vi "open dataset.vi"(9 "old dataset":T1) -> (1 "new dataset":T1)   [LabVIEW 2025]
panel:
  # "Load or Save dataset. \nDataset includes raw data, data names, scales, show/hide indices parameters."
  # "On: Scale parameters defined by 'scaling' function will be used."
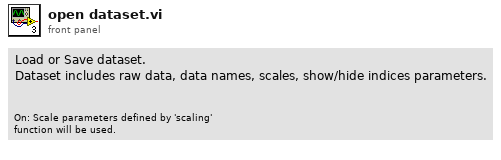
[diagram p1: front panel]
types:
  T1 = cluster{"data cluster":cluster{"all data":dbl[][]}[], "Scale":u16, "scale matrix":dbl[][], "universal y-scale":dbl, "data names":string[], "new dataset?":bool, "show files 2":cluster{"String":string, "Boolean":bool, "begin":u32, "length":u32, "y weight":dbl}[]}
  T2 = enum16{"Left Button", "Center Button", "Right Button", "Window Close"}
  T3 = cluster{"String":string, "Boolean":bool, "begin":u32, "length":u32, "y weight":dbl}[]
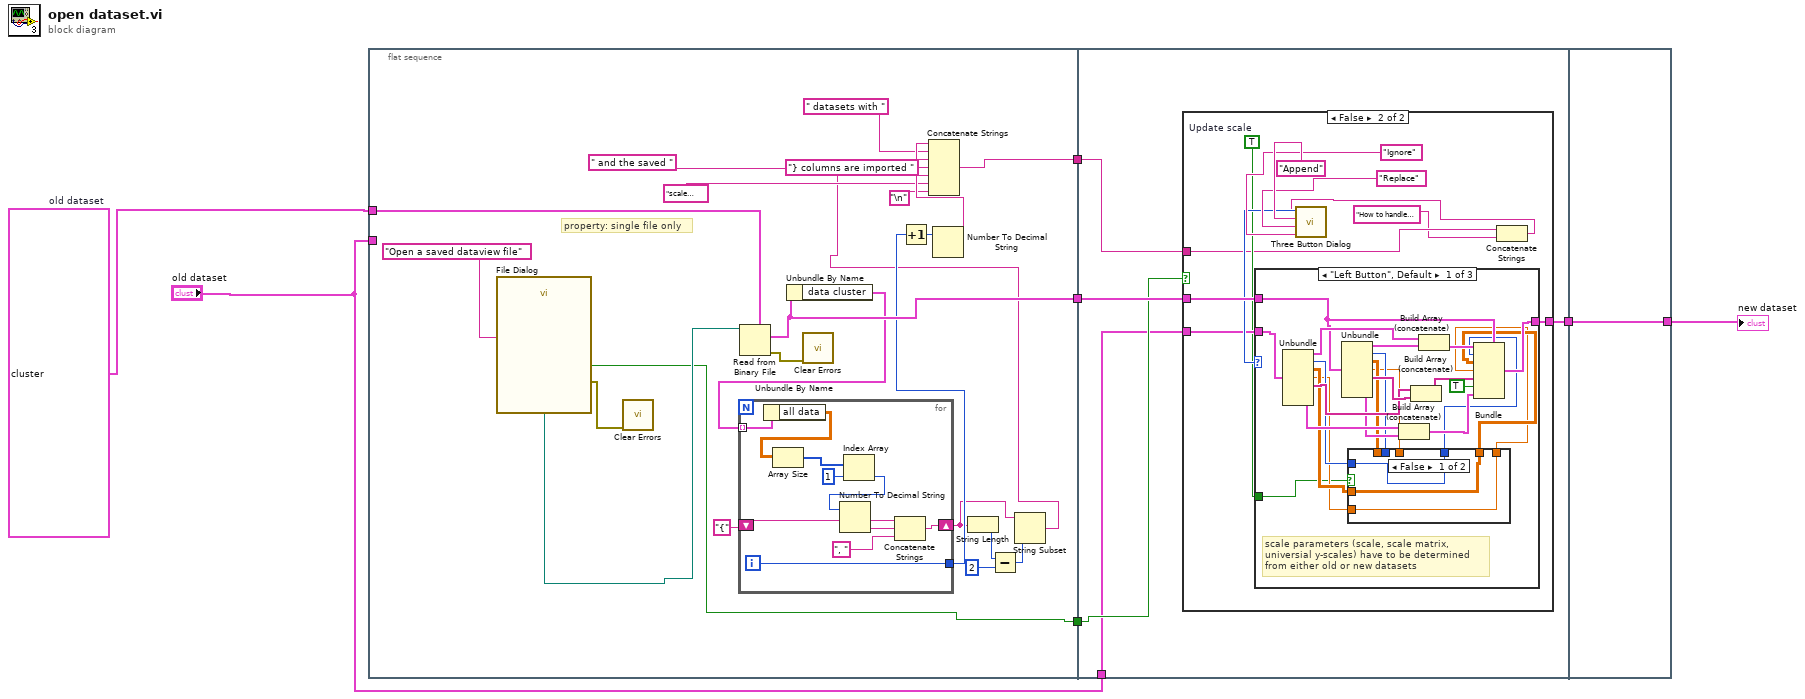
[diagram p0: block diagram]
diagram:
  w6 = T1 {"data cluster"=[{"all data"=array60x36[2160 elements]}], "Scale"=0, "scale matrix"=[], "universal y-scale"=1.0, "data names"=["FGT512para_PPMS_Hsweep_170K3.dat"], "new dataset?"=TRUE, "show files 2"=[]}  # old dataset
  n1 = flat-sequence {
    tunnel: [w19] -> w5
    tunnel: [w28] -> w4
    tunnel: "old dataset" -> [_]
    tunnel: w6 -> [w27]
    tunnel: [w20] -> w2
    tunnel: w5 -> [w45]
    tunnel: "old dataset" -> [w42]
    tunnel: [w44] -> w3
    tunnel: w4 -> [w43]
    tunnel: w2 -> [w41]
    tunnel: [w89] -> w1
    tunnel: w3 -> [w89]
    frame #0 {
      # "property: single file only"
      n2 = call "File Dialog"("prompt"="Open a saved dataview file") -> ("selected path"=w29:path, "cancelled"=w28:bool, "error out"=w30:errorcluster)  [unwired: 11 in, 1 out]
      n3 = call <vilib>:"Clear Errors.vi"("error in (no error)"=w30) -> ()  [unwired: 5 in, 2 out]
      n4 = Read from Binary File(5:w27, 11:w29) -> (0:w26:errorcluster, 2:w19:T1)  [unwired: 4 in, 2 out]
      n5 = Unbundle By Name(w19) -> ("data cluster"=w18:cluster{"all data":dbl[][]}[])
      n6 = for {
        tunnel: w18 -> [w38] mode=indexing
        tunnel: [w36] -> w17
        shift-right: [w31] -> w12
        shift-left: "{" -> [w34]
        i -> [w36]
        n7 = Unbundle By Name(w38) -> ("all data"=w37:dbl[][])
        n8 = Array Size(array=w37) -> (size(s)=w40:i32[])
        n9 = Index Array(array=w40, index=1) -> (element=w35:i32)
        n10 = Number To Decimal String(number=w35) -> (decimal integer string=w33:string)  [unwired: 1 in]
        n11 = Concatenate Strings(w34, w33, ", " ("string")) -> (w31:string)
      }
      n12 = call <vilib>:"Clear Errors.vi"("error in (no error)"=w26) -> ()  [unwired: 5 in, 2 out]
      n13 = Increment(x=w17) -> (x+1=w16:i32)
      n14 = Number To Decimal String(number=w16) -> (decimal integer string=w24:string)  [unwired: 1 in]
      n15 = String Length(string=w12) -> (length=w10:i32)
      n16 = Subtract(x=w10, y=2) -> (x-y=w8:i32)
      n17 = String Subset(string=w12, length (rest)=w8) -> (substring=w11:string)  [unwired: 1 in]
      n18 = Concatenate Strings(w24, " datasets with " ("string"), w11, "} columns are imported " ("string"), " and the saved " ("Center Button Text (\"No\")"), "scale parameters will be used." ("string"), "\n") -> (w20:string)
    }
    frame #1 {
      n19 = case shown="False" w43 {
        tunnel: w45 -> [_ w54]
        tunnel: [w46 w53] -> w44
        tunnel: w42 -> [w46 w51]
        tunnel: w41 -> [_ w48]
        frame True {
        }
        frame False {
          w49 = TRUE  # Update scale
          n20 = Concatenate Strings(w48, "How to handle the loaded datasets?" ("message")) -> (w50:string)
          n21 = call <vilib>:"Three Button Dialog.vi"("Right Button Text (\"Cancel\")"="Ignore" ("Right Button Text (\"Cancel\")"), "Center Button Text (\"No\")"="Replace" ("Center Button Text (\"No\")"), "Left Button Text (\"Yes\")"="Append" ("Left Button Text (\"Yes\")"), "message"=w50) -> ("Which Button?"=w52:T2)  [unwired: 7 in]
          n22 = case shown="\"Left Button\", Default" w52 {
            tunnel: [w69 w87 w88] -> w53
            tunnel: w54 -> [w73 w87 _]
            tunnel: w51 -> [w80 _ w88]
            tunnel: w49 -> [w58 _ _]
            frame "Left Button", Default {
              # "scale parameters (scale, scale matrix, \nuniversial y-scales) have to be determined\nfrom either old or new datasets"
              n23 = Unbundle(w80) -> ("data cluster"=w79:cluster{"all data":dbl[][]}[], "Scale"=w61:u16, "scale matrix"=w60:dbl[][], "universal y-scale"=w59:dbl, "data names"=w75:string[], "show files 2"=w71:T3)  [unwired: 1 out]
              n24 = Unbundle(w73) -> ("data cluster"=w78:cluster{"all data":dbl[][]}[], "Scale"=w66:u16, "scale matrix"=w64:dbl[][], "universal y-scale"=w62:dbl, "data names"=w76:string[], "show files 2"=w70:T3)  [unwired: 1 out]
              n25 = case shown="False" w58 {
                tunnel: [w83 w86] -> w67
                tunnel: w66 -> [_ w86]
                tunnel: [w82 w85] -> w65
                tunnel: w64 -> [_ w85]
                tunnel: [w81 w84] -> w63
                tunnel: w62 -> [_ w84]
                tunnel: w61 -> [w83 _]
                tunnel: w60 -> [w82 _]
                tunnel: w59 -> [w81 _]
                frame False {
                }
                frame True {
                }
              }
              n26 = Build Array (concatenate)(w71, w70) -> (w68:T3)
              n27 = Build Array (concatenate)(w75, w76) -> (w74:string[])
              n28 = Build Array (concatenate)(w79, w78) -> (w77:cluster{"all data":dbl[][]}[])
              n29 = Bundle(cluster=w73, "data cluster"=w77, "Scale"=w67, "scale matrix"=w65, "universal y-scale"=w63, "data names"=w74, "new dataset?"=TRUE, "show files 2"=w68) -> (w69:T1)
            }
            frame "Center Button" {
            }
            frame "Right Button" {
            }
          }
        }
      }
    }
    frame #2 {
    }
  }
  "new dataset" <- w1
